vi "ROS_Close_Topics.vi"(8 "error in (no error)":errorcluster, 11 "ROS_In_Array":T1[](array[typedef])) -> (0 "error out":errorcluster)   [LabVIEW 2017]
doc: "Close ROS topics"
uses:
  <vilib>/Tufts CEEO ROS for LabVIEW Software/ROS/Code/SubVIs/_ROSControl.ctl
  <vilib>/Tufts CEEO ROS for LabVIEW Software/ROS/Code/SubVIs/_ROSDirection.ctl
  <vilib>/Tufts CEEO ROS for LabVIEW Software/ROS/MessageBuilding/std_msgs/subs/float32Scalar.vi
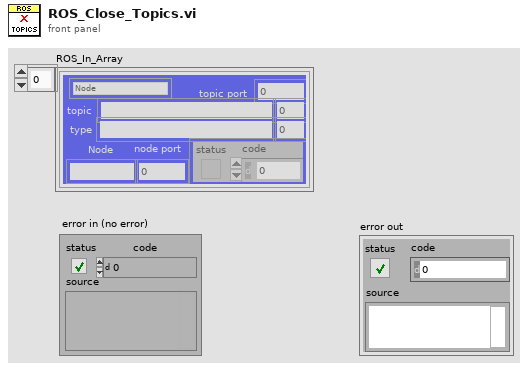
[diagram p1: front panel]
types:
  T1 = typedef "_ROSControl.ctl" = cluster{"topic port":u16, "Node":string, "topic":string, "type":string, "node port":u16, "error ":errorcluster, "Direction":T2, "Update (ms)":u16, "FIFO size":u16}
  T2 = typedef "_ROSDirection.ctl" = enum16{"Node", "Publisher", "Subscriber", "ServiceClient", "ServiceProvider"}
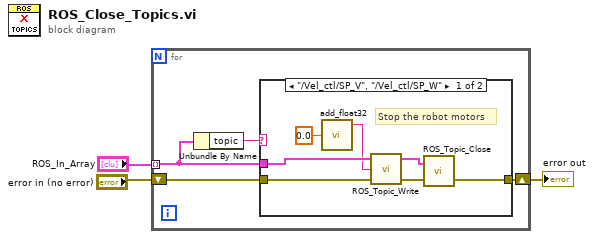
[diagram p0: block diagram]
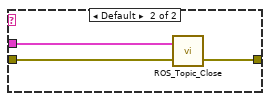
[diagram p2: hidden frame]
diagram:
  n1 = for {
    tunnel: "ROS_In_Array" -> [w5] mode=indexing
    shift-right: [w7] -> w1
    shift-left: "error in (no error)" -> [w6]
    n2 = Unbundle By Name(w5) -> ("topic"=w4:string)
    n3 = case shown="\"/Vel_ctl/SP_V\", \"/Vel_ctl/SP_W\"" w4 {
      tunnel: w5 -> [w11 w17]
      tunnel: [w14 w16] -> w7
      tunnel: w6 -> [w13 w15]
      frame "/Vel_ctl/SP_V", "/Vel_ctl/SP_W" {
        # "Stop the robot motors"
        n4 = call-poly <vilib>:"add_float32.vi"("Numeric"=sgl 0.0) -> ("msg out"=w9:string)  [unwired: 4 in]
        n5 = call <vilib>:"ROS_Topic_Write.vi"("error in (no error)"=w13, "Msg in"=w9, "ROS in"=w11) -> ("error out"=w12:errorcluster, "ROS out"=w10:T1)  [unwired: 1 in]
        n6 = call <vilib>:"ROS_Topic_Close.vi"("error in"=w12, "ROS in"=w10) -> ("error out"=w14:errorcluster)  [unwired: 2 in]
      }
      frame Default {
        n7 = call <vilib>:"ROS_Topic_Close.vi"("error in"=w15, "ROS in"=w17) -> ("error out"=w16:errorcluster)  [unwired: 2 in]
      }
    }
  }
  "error out" <- w1
